vi "finish collecting results.vi"(8 "error in (no error)":errorcluster, 10 "psqlite":refnum<class "sqlite3.lvclass">, 11 "active statement in":T1={"ppStmt"=0, "column count"=0, "bind offset"=1, "bind param count"=1, "finished?"=FALSE, "column offset"=0, "column types"=[]} {"column types" items=["INTEGER"=1, "FLOAT"=2, "STRING"=3, "BLOB"=4, "NULL"=5]}) -> (0 "error out":errorcluster, 3 "active statement out":T1={"ppStmt"=0, "column count"=0, "bind offset"=1, "bind param count"=1, "finished?"=FALSE, "column offset"=0, "column types"=[]} {"column types" items=["INTEGER"=1, "FLOAT"=2, "STRING"=3, "BLOB"=4, "NULL"=5]})   [LabVIEW 2014, in "SQLite3LV.lvlib" / "cursor.lvclass"]
uses:
  cursor.lvclass
  ctl_active_statement.ctl
  SQLite3 Class/sqlite3.lvclass
  SQLite3LV.lvlib
  sqlite3_64.dll
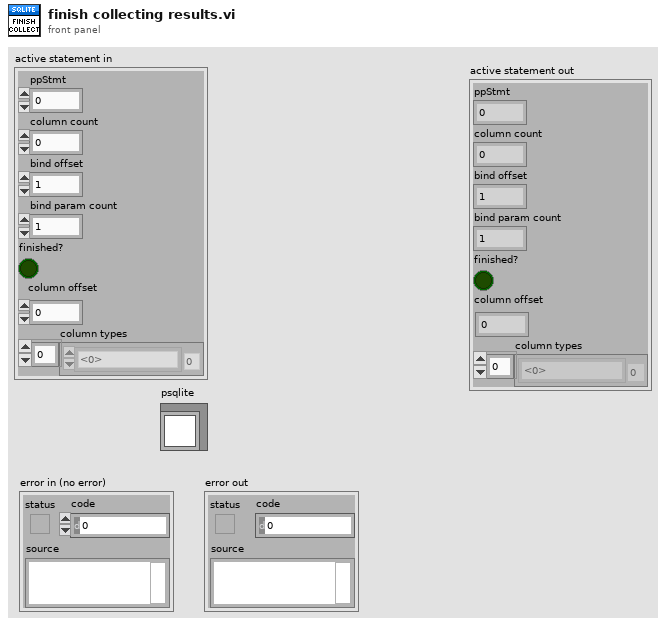
[diagram p1: front panel]
types:
  T1 = typedef "SQLite3LV.lvlib/cursor.lvclass/ctl_active_statement.ctl" = cluster{"ppStmt":i64, "column count":i32, "bind offset":i32, "bind param count":i32, "finished?":bool, "column offset":i32, "column types":i32[]}
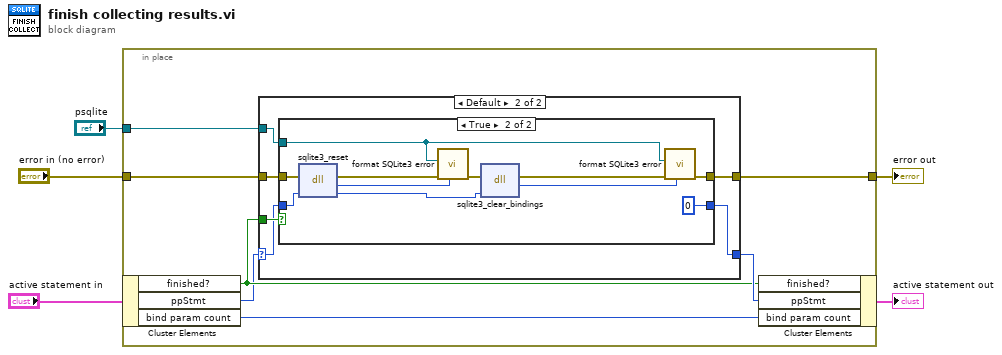
[diagram p0: block diagram]
diagram:
  n1 = in-place {
    in-place-border: "error in (no error)" -> [w12]
    in-place-border: "psqlite" -> [w11]
    in-place-border: [w10] -> w3
    n2 = in-place-cluster #1("active statement in") -> ("finished?"=w8:bool, "ppStmt"=w7:i64, "bind param count"=w6:i32)
    n3 = case shown="Default" w7 {
      selector: w7 -> [w14 w15]
      tunnel: w12 -> [w13 w20]
      tunnel: w11 -> [_ w19]
      tunnel: [w13 w18] -> w10
      tunnel: [w14 w17] -> w9
      tunnel: w8 -> [_ w16]
      frame 0 {
      }
      frame Default {
        n4 = case shown="True" w16 {
          tunnel: w20 -> [w22 w33]
          tunnel: w19 -> [_ w32]
          tunnel: [w22 w31] -> w18
          tunnel: [w21 i64 0 ("ppStmt")] -> w17
          tunnel: w15 -> [w21 w29]
          frame False {
          }
          frame True {
            n5 = dll-call lib="C:/Users/BobUser/Desktop/LVTables/sqlite3**.*" fn="sqlite3_reset"(error in=w33, "pStmt"=w29) -> (error out=w26:errorcluster, "result code"=w27:i32, "pStmt"=w28:i64)  [unwired: 2 in, 1 out]
            n6 = call "format SQLite3 error.vi"("SQLite3LV Connection result"=w27, "error in (no error)"=w26, "psqlite"=w32) -> ("error out"=w25:errorcluster)  [unwired: 8 in]
            n7 = dll-call lib="C:/Users/BobUser/Desktop/LVTables/sqlite3**.*" fn="sqlite3_clear_bindings"(error in=w25, "pStmt"=w28) -> (error out=w24:errorcluster, "result code"=w23:i32)  [unwired: 3 in, 1 out]
            n8 = call "format SQLite3 error.vi"("SQLite3LV Connection result"=w23, "error in (no error)"=w24, "psqlite"=w32) -> ("error out"=w31:errorcluster)  [unwired: 8 in]
          }
        }
      }
    }
    n9 = in-place-cluster #1("finished?"=w8, "ppStmt"=w9, "bind param count"=w6) -> (→"active statement out":T1)
  }
  "error out" <- w3
